vi "Main.vi"() -> ()   [LabVIEW 2013]
doc: "This template is for the Queued Message Handler design pattern.\n\nThe Event Handling Loop generates messages based on user interface actions.\n\nThe Message Handling Loop processes messages generated by the Event Handling Loop, or by other messages. The messages are string values, so new messages can be added easily to the Message Cases case structure in the Message Handling Loop. Each message cluster can also provide an optional value for Message Data, which is a variant that can be converted to whatever message-specific data is required."
uses:
  <vilib>/vision/Image Controls.llb/IMAQ Image.ctl
  Image Processing/Mask ROI FG Enum.ctl
  Message Passing/MsgQ Loops enum.ctl
  System Status/Status FG Enum.ctl
  Globals/Average Sector Data.vi
  controls/UI Data.ctl
  Message Queue/Message Queue.lvlib
  User Event - Stop/User Event - Stop.lvlib
  FPGA/FPGA Frame Grabbing.lvlib
  Image Processing/Image Processing.lvlib
  Common/State Machines/State Machine Lib.lvlib
  Message Passing/Main MsgQ.lvlib
  Common/GUI/GUI.lvlib
  <vilib>/rvi/interface/nirviReadWriteControl/nirviReadWriteControl.xnode
  FGs/FPGA_Reference.ctl
  FPGA Bitfiles/WBA256SectorsSim_FPGATargetSim.lvbitx
  <vilib>/rvi/errors/niLvFpgaMergeErrorWithErrorCode.vi
  NiFpgaLv.dll
  <vilib>/rvi/errors/niLvFpgaAdjustHostInterfaceError.vi
panel:
  out "Frame Count":u16
  out "Frames Acquired":u32
  in  "Disable Background Subtraction":bool
  out "Analysis Ticks":u32
  out "Accumulate Ticks":u32
  out "FPGA Display Image":T1(plugin-control)
  out "Right Wingbeat Avg Graph":u8[](graph)
  in  "Start Serial Server":bool=TRUE
  out "Left Wingbeat Avg Graph":u8[](graph)
  in  "Stop Charts":bool
  in  "Wing ROIs":T2
  out "FPGA image info":T5={"Image Type"=0, "Unit"=enum."Undefined", "X Resolution"=2040, "Y Resolution"=1088, "X Step"=1.0, "Y Step"=1.0, "Image Name"="Image"} {"Image Type" items=["Grayscale (U8)", "Grayscale (I16)", "Grayscale (SGL)", "Complex (CSG)", "RGB (U32)", "HSL (U32)", "RGB (U64)", "Grayscale (U16)"]}
  in  "Stream?":bool
  out "FPGA Image":T1
  in  "Test Visual Response":bool
  in  "Test FPGA":bool
  out "Status Update":string="VI Stopped"
  in  "Define Mask":bool
  in  "Acquire Image":bool
  in  "Stop":bool
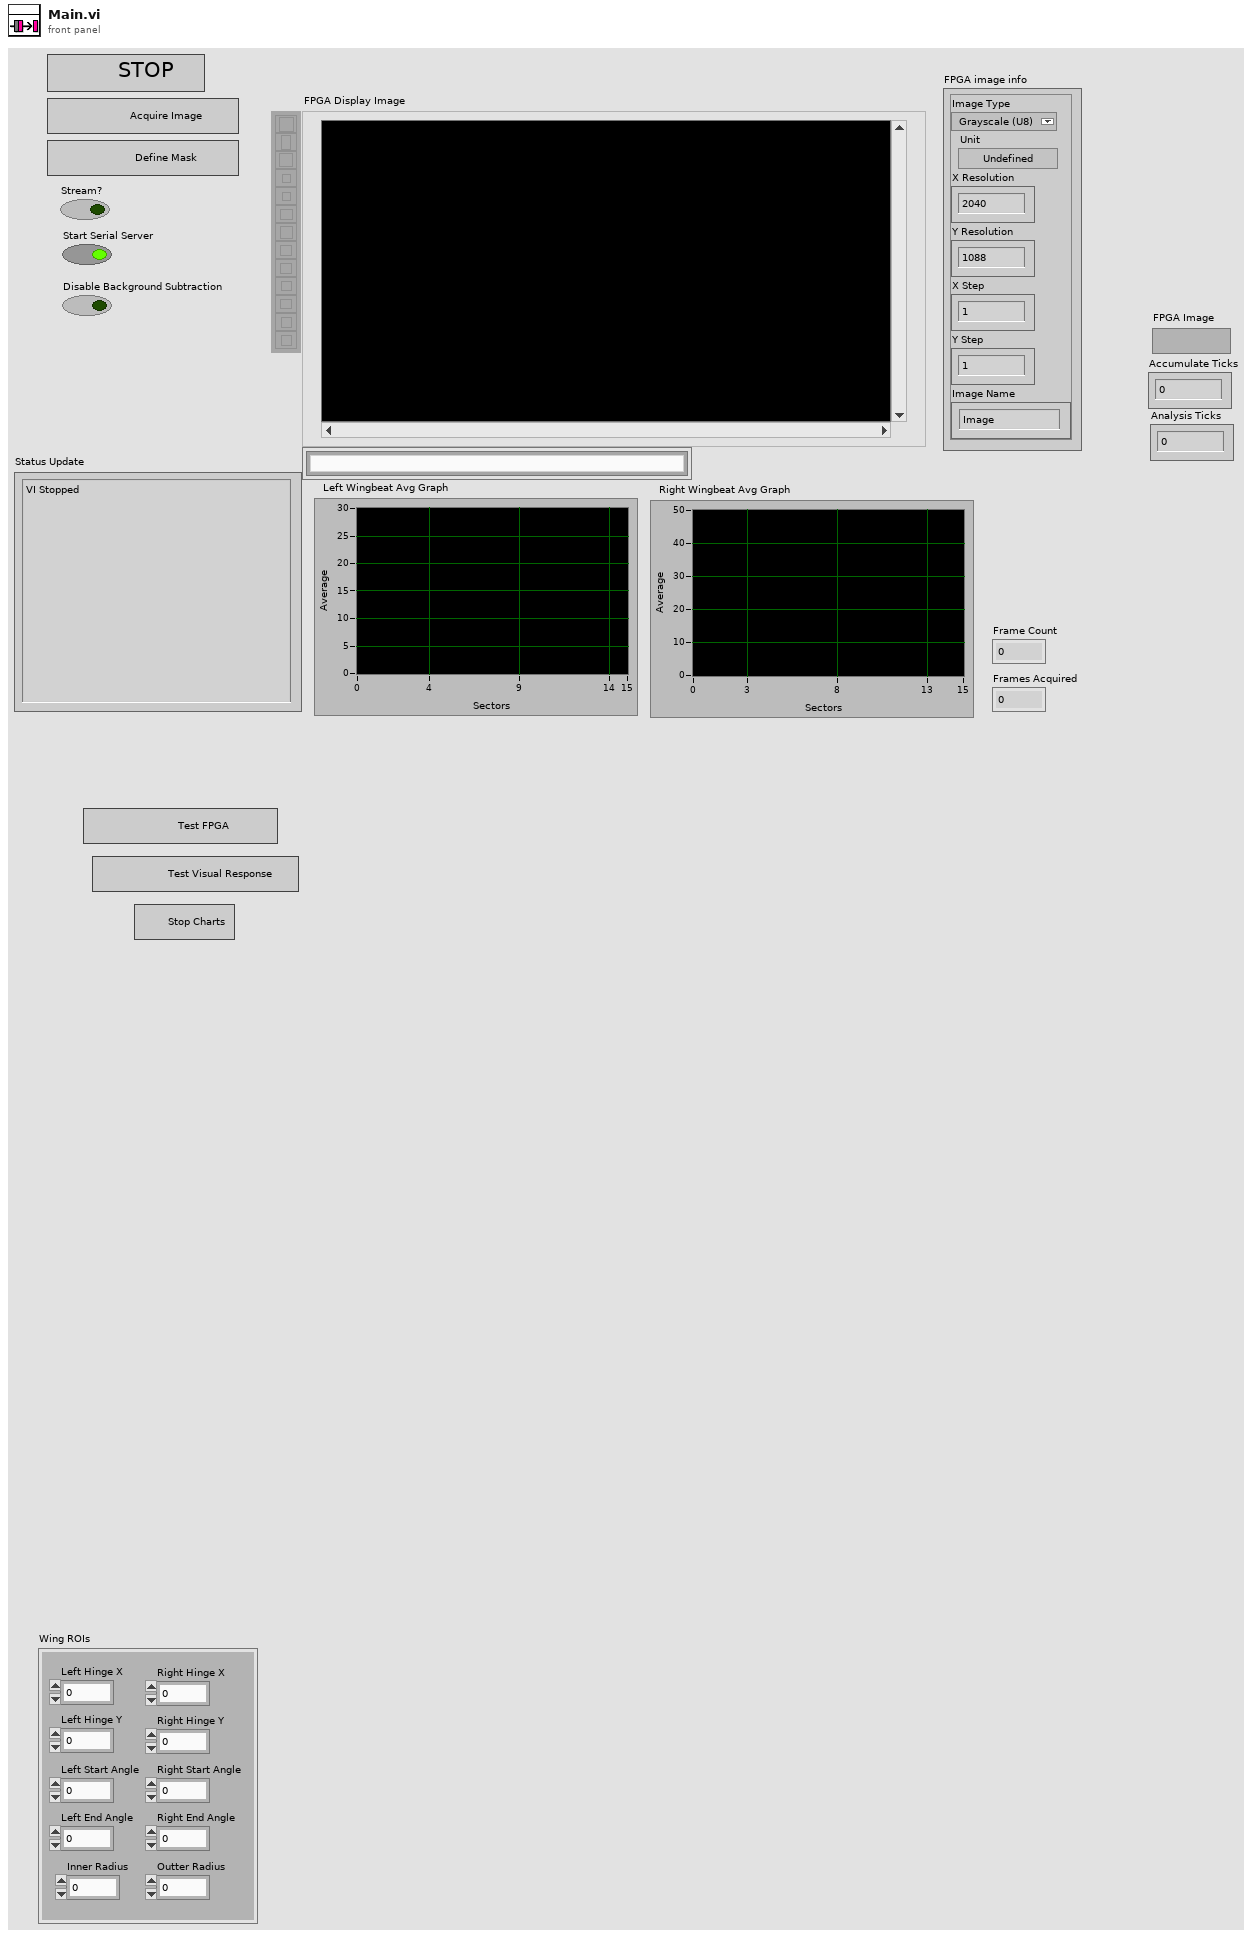
[diagram p1: front panel]
types:
  T1 = typedef "IMAQ Image.ctl" = refnum<image>
  T2 = cluster{"Left Hinge X":u16, "Left Hinge Y":u16, "Inner Radius":u16, "Outter Radius":u16, "Right Hinge X":u16, "Right Hinge Y":u16, "Right Start Angle":i16, "Right End Angle":i16, "Left Start Angle":i16, "Left End Angle":i16}
  T3 = typedef "Image Type" = u32
  T4 = typedef "Image Unit" = enum32{"Undefined", "Angström", "Micrometer", "Millimeter", "Centimeter", "Meter", "Kilometer", "Microinch", "Inch", "Feet", "Nautical miles", "Standard miles", "Steps"}
  T5 = cluster{"Image Type":T3, "Unit":T4, "X Resolution":i32, "Y Resolution":i32, "X Step":sgl, "Y Step":sgl, "Image Name":string}
  T6 = typedef "State Machine Lib.lvlib/STATE cluster.ctl" = cluster{"State":string, "Parameters":variant}
  T7 = typedef "Main MsgQ.lvlib/MsgQ Loops enum.ctl" = enum16{"User Interface", "Image Acq"}
  T8 = typedef "Mask ROI FG Enum.ctl" = enum16{"Read", "Write", "Enable Background", "Disable Background"}
  T9 = typedef "Status FG Enum.ctl" = enum16{"Reset", "Read", "Write"}
  T10 = typedef "FPGA_Reference.ctl" = refnum<k20>
  T11 = typedef "Mask ROI Cluster.ctl" = cluster{"left annulus":T12, "right annulus":T12, "Threshold Range":cluster{"Lower value":dbl, "Upper value":dbl}, "[Avg BG]":u8[], "Number of Sectors":u8, "Left ROI":T13, "Right ROI":T13, "Left Start Angle Duty Cycle":fxp<+,8,0>, "Left End Angle Duty Cycle":fxp<+,8,0>, "Right End Angle Duty Cycle":fxp<+,8,0>, "Right Start Angle Duty Cycle":fxp<+,8,0>, "[Sector ROIs]":T13[]}
  T12 = typedef "IMAQ Circle" = cluster{"Center X":i32, "Center Y":i32, "Inner Radius":i32, "Outer Radius":i32, "Start Angle":dbl, "End Angle":dbl}
  T13 = typedef "ROI Descriptor" = cluster{"Global Rectangle":i32[], "Contours":cluster{"ID":enum32{"External", "Internal"}, "Type":u32, "Coordinates":i32[]}[]}
  T14 = typedef "UI Data.ctl" = cluster{"Boolean <Replace Me>":bool, "Initial Message":string, "Numeric <Replace Me>":dbl, "Acquire Image Ref":refnum<vi>, "Define Mask Ref":refnum<vi>, "Status Update Ref":refnum<vi>, "Stop Button Ref":refnum<vi>, "FPGA Image":T1, "Processed Image":T1, "Left Annulus":cluster{"Center X":i32, "Center Y":i32, "Inner Radius":i32, "Outer Radius":i32, "Start Angle":dbl, "End Angle":dbl}, "Right Annulus":cluster{"Center X":i32, "Center Y":i32, "Inner Radius":i32, "Outer Radius":i32, "Start Angle":dbl, "End Angle":dbl}}
  T15 = typedef "Message Queue.lvlib/All Message Queues.ctl" = cluster{"UI":refnum<queue>}
  T16 = cluster{"Center X":i32, "Center Y":i32, "Inner Radius":i32, "Outer Radius":i32, "Start Angle":dbl, "End Angle":dbl}
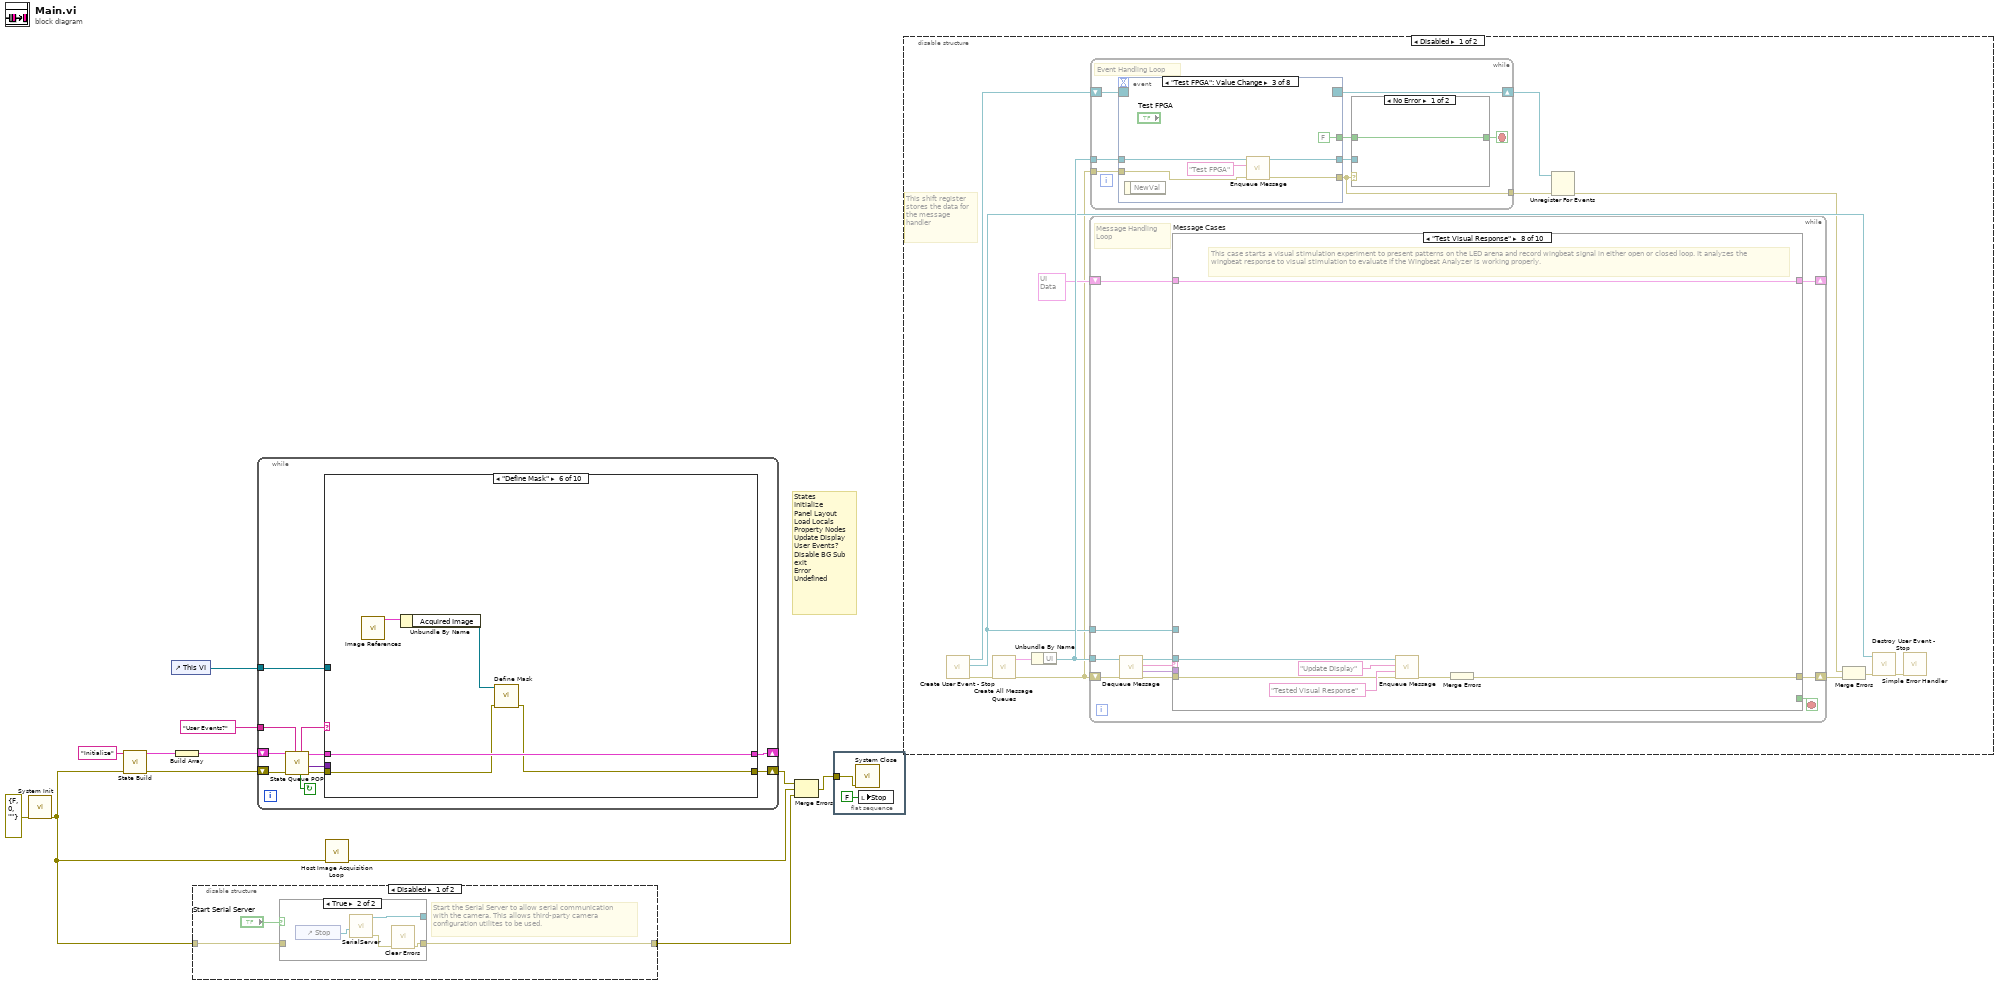
[diagram p0: block diagram]
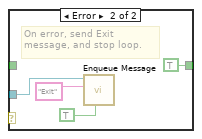
[diagram p4: hidden frame]
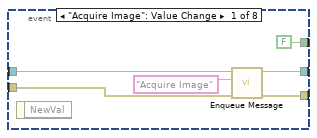
[diagram p5: hidden frame]
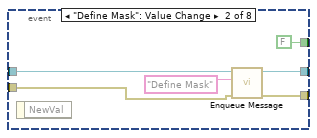
[diagram p6: hidden frame]
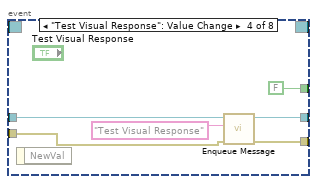
[diagram p7: hidden frame]
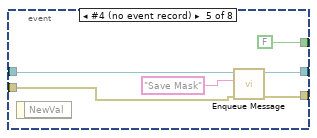
[diagram p8: hidden frame]
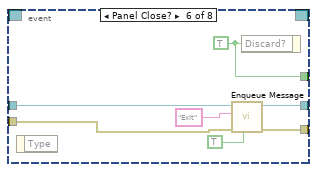
[diagram p9: hidden frame]
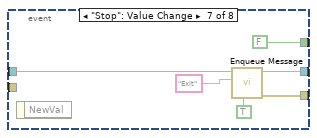
[diagram p10: hidden frame]
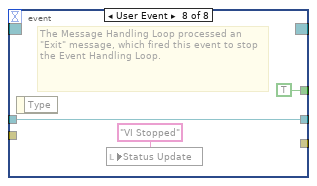
[diagram p11: hidden frame]
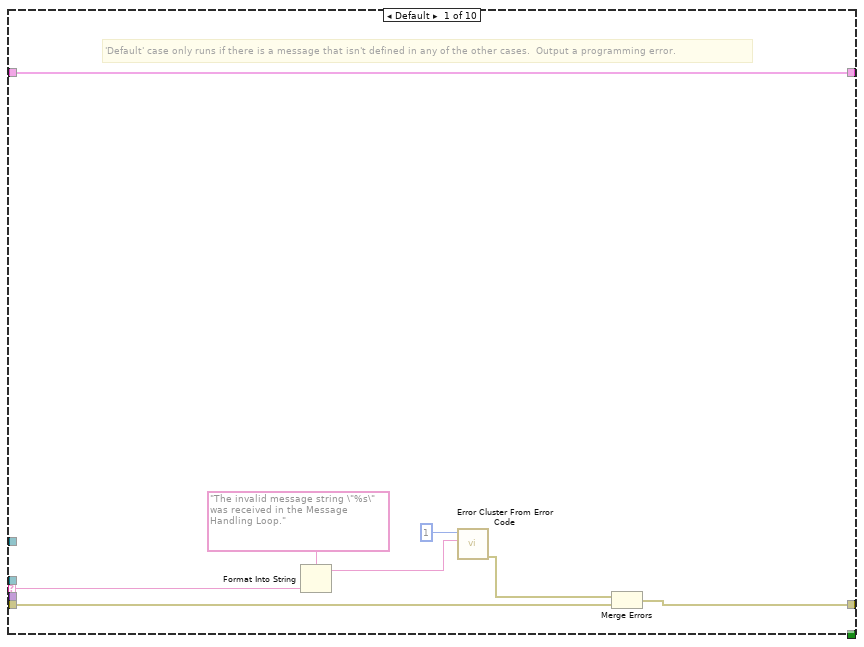
[diagram p12: hidden frame]
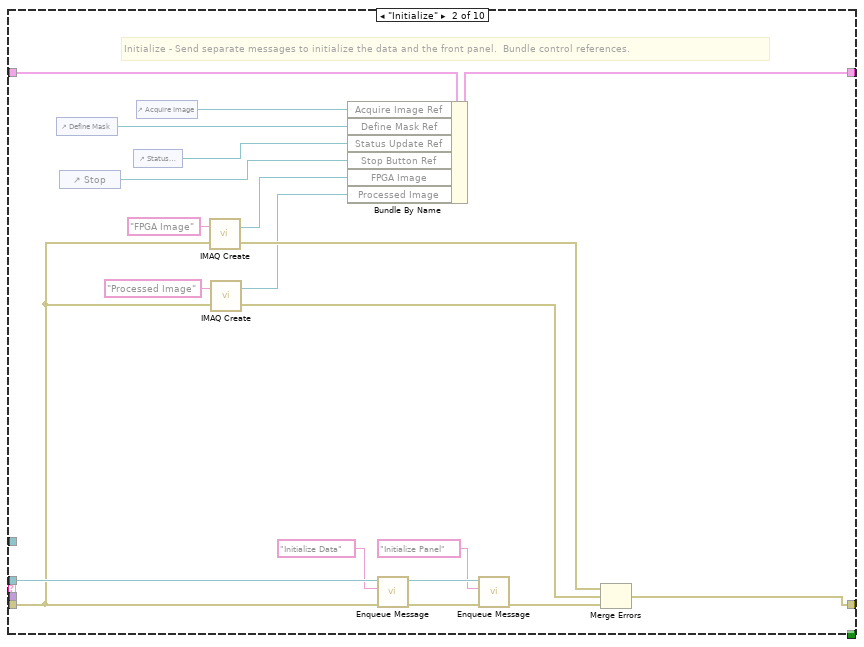
[diagram p13: hidden frame]
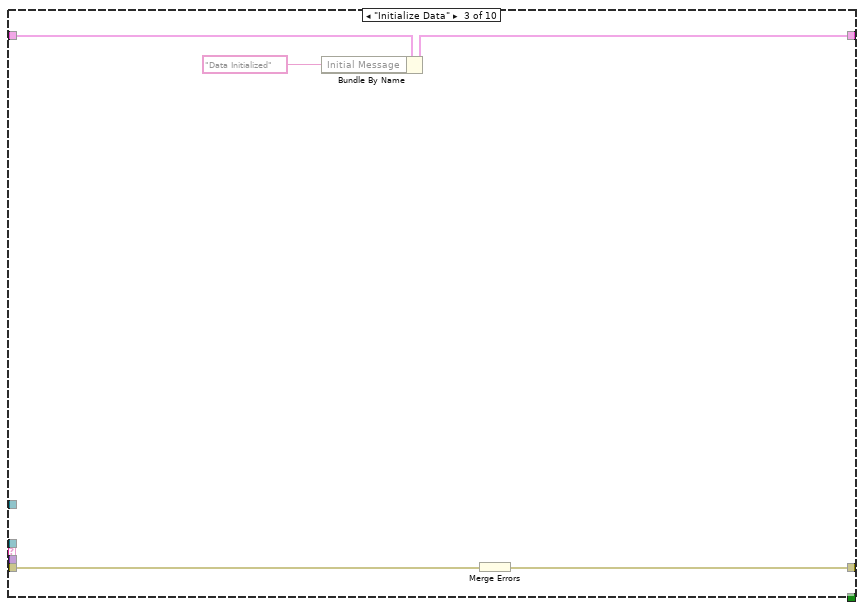
[diagram p14: hidden frame]
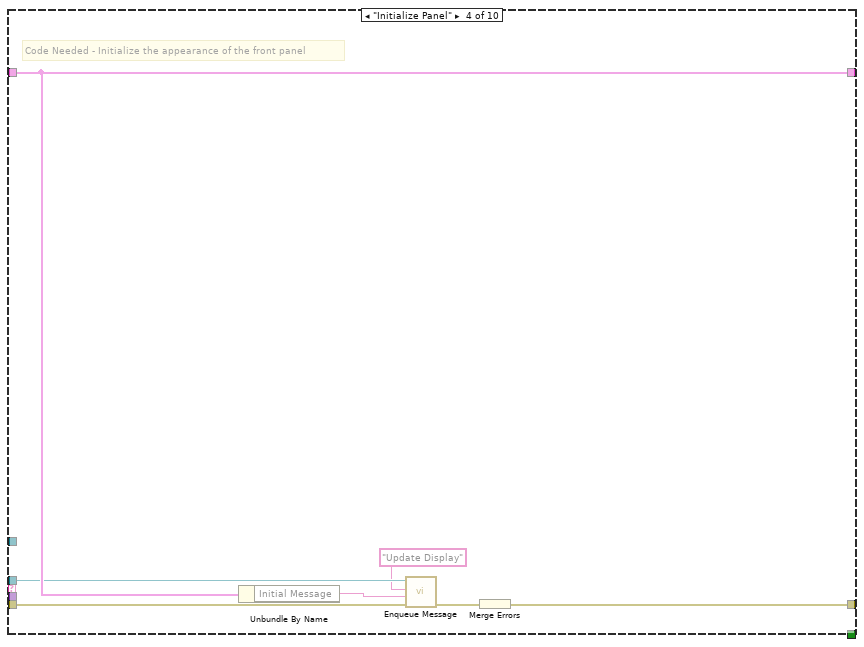
[diagram p15: hidden frame]
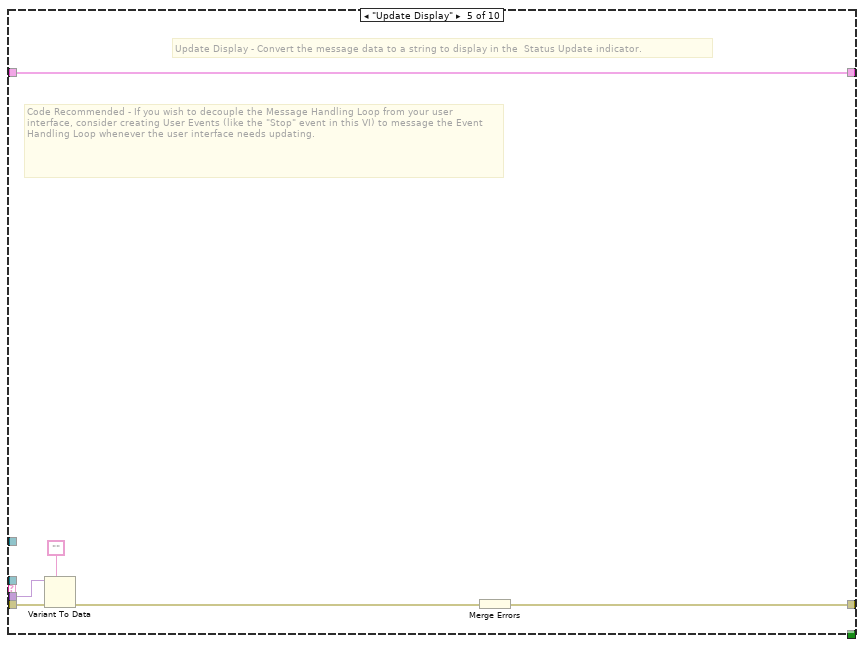
[diagram p16: hidden frame]
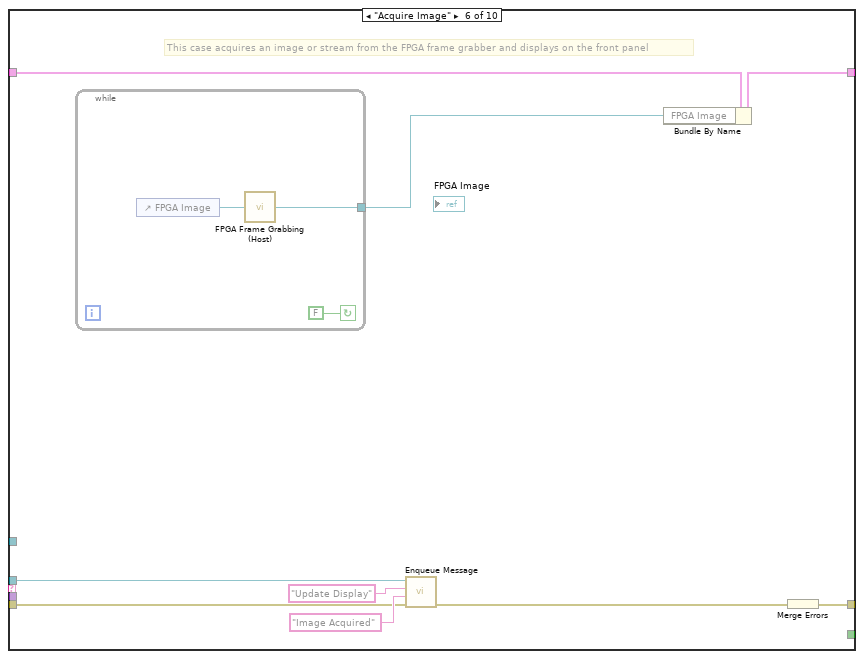
[diagram p17: hidden frame]
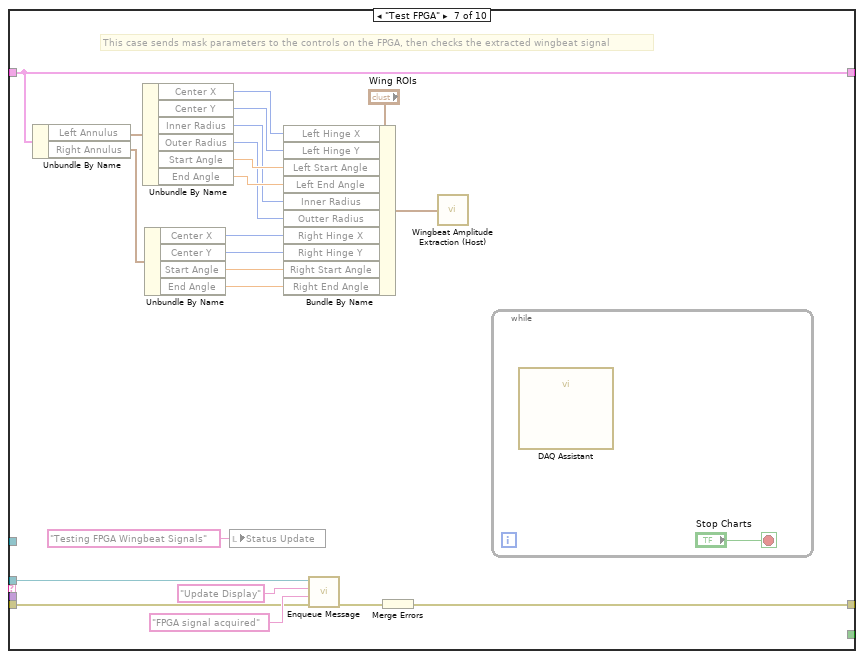
[diagram p18: hidden frame]
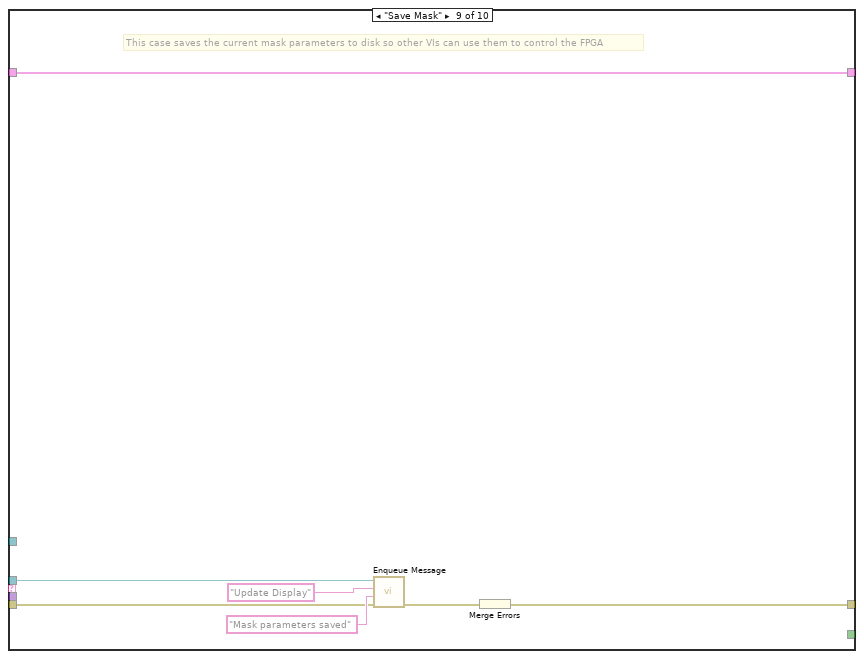
[diagram p19: hidden frame]
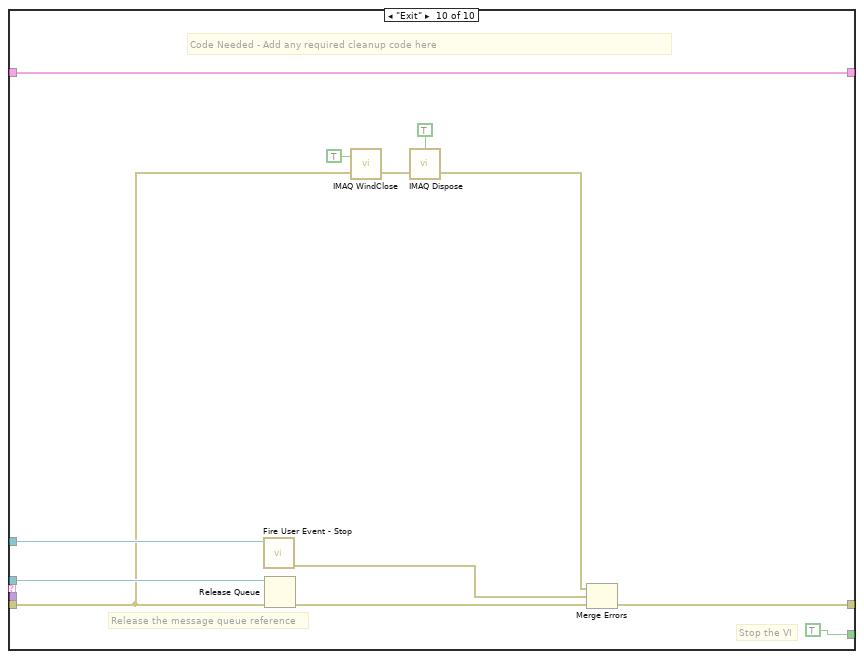
[diagram p20: hidden frame]
diagram:
  # "States\nInitialize\nPanel Layout\nLoad Locals\nProperty Nodes\nUpdate Display\nUser Events?\nDisable BG Sub\nexit\nError\nUndefined"
  n1 = call "System Init.vi"("error in (no error)"=errorcluster {"status"=FALSE, "code"=0, "source"=""}) -> ("error out"=w11:errorcluster)  [unwired: 10 in]
  n2 = call "State Build.vi"("error in (no error)"=w11, "State"="Initialize") -> ("error out"=w7:errorcluster, "State Out"=w9:T6)  [unwired: 8 in]
  n3 = control-ref of="This VI"() -> (w5:refnum<vi>)
  n4 = Build Array(w9) -> (w8:T6[])
  n5 = disable-structure shown="Disabled" {
    disable-tunnel: w11 -> [w14 w21]
    disable-tunnel: [w13 w21] -> w1
    frame Disabled {
      # "Start the Serial Server to allow serial communication\nwith the camera. This allows third-party camera\nconfiguration utilites to be used."
      n6 = case shown="True" "Start Serial Server" {
        tunnel: [_ w20] -> _
        tunnel: w14 -> [w16 _]
        tunnel: [w16 w18] -> w13
        frame False {
        }
        frame True {
          n7 = control-ref of="Stop"() -> (w19:refnum<vi>)
          n8 = call "SerialServer.vi"("Stop Refnum"=w19) -> ("error out"=w17:errorcluster, "FPGA VI Reference Out"=w20:refnum<k20>)  [unwired: 5 in]
          n9 = call <vilib>:"Clear Errors.vi"("error in (no error)"=w17) -> ("error out"=w18:errorcluster)  [unwired: 6 in]
        }
      }
    }
    frame Enabled {
    }
  }
  n10 = while {
    shift-right: [w26] -> _
    shift-left: w8 -> [w32]
    shift-right: [w24] -> w4
    shift-left: w7 -> [w31]
    tunnel: "User Events?" ("State") -> [w29]
    tunnel: w5 -> [w27]
    stop <- w30 continue-if-true
    n11 = call "State Queue POP.vi"("Default state"=w29, "error in (no error)"=w31, "State que in"=w32) -> ("error out"=w23:errorcluster, "Parameters"=w22:variant, "State que out"=w25:T6[], "Not Exit?"=w30:bool, "State case out"=w28:string)  [unwired: 4 in]
    n12 = case shown="\"Define Mask\"" w28 {
      tunnel: w27 -> [_ _ w43 _ _ _ _ _ _ _]
      tunnel: [w34 w35 w40 w46 w48 w53 w54 w71 w112 w140] -> w26
      tunnel: w25 -> [w34 w38 w40 w46 w48 w53 w54 w70 _ w140]
      tunnel: [w33 w36 w41 w45 w47 w51 w55 w69 w111 w138] -> w24
      tunnel: w23 -> [w33 w37 w42 w45 w47 w52 w66 w68 w113 w122]
      tunnel: w22 -> [_ _ _ _ _ _ w65 w67 _ _]
      frame Default {
      }
      frame "Initialize" {
        n13 = call "State Queue PUSH multiple states no parameters.vi"("States to queue"=string[] ["Panel Layout", "Load Locals", "Property Nodes", "Update Display"], "error in (no error)"=w37, "State que in"=w38) -> ("error out"=w36:errorcluster, "State que out"=w35:T6[])  [unwired: 7 in]
      }
      frame "Panel Layout" {
        # "Reset origin to 0,0"
        n14 = call "Reset all pane origins.vi"("error in (no error"=w42, "Vi Ref In"=w43) -> ("error out"=w41:errorcluster)  [unwired: 8 in, 1 out]
      }
      frame "Load Locals" {
        w44 = FALSE ("Stream?")
        n15 = local write "Stream?"(w44) -> ()
        n16 = local write "Disable Background Subtraction"(w44) -> ()
      }
      frame "Property Nodes" {
      }
      frame "Define Mask" {
        n17 = call "Image References.vi"() -> ("Images"=w50:cluster{"Acquired Image":T1, "Display Image":T1})  [unwired: 10 in, 1 out]
        n18 = Unbundle By Name(w50) -> ("Acquired Image"=w49:T1)
        n19 = call "Define Mask.vi"("error in (no error)"=w52, "FPGA Image"=w49) -> ("error out"=w51:errorcluster)  [unwired: 9 in]
      }
      frame "Disable BG Sub" {
        n20 = Variant To Data(error in=w66, type=FALSE, Variant=w65) -> (data=w63:bool, error out=w60:errorcluster)
        n21 = Select(t=Mask_ROI_FG_Enum."Disable Background" ("Operation"), s=w63, f=Mask_ROI_FG_Enum."Enable Background" ("Operation")) -> (s? t:f=w59:T8)
        n22 = call "Mask ROI FG.vi"("error in (no error)"=w60, "Operation"=w59) -> ("error out"=w56:errorcluster)  [unwired: 8 in, 1 out]
        n23 = call "Send MsgQ.vi"("error in (no error)"=w56, "Message String"="Update Sector Parameters", "Send to MsgQ"=MsgQ_Loops_enum."Image Acq") -> ("error out"=w55:errorcluster)  [unwired: 8 in]
      }
      frame "User Events?" {
        n24 = event shown="[1] \"Acquire Image\": Value Change" {
          selector: _ -> [_ _ _ _ _ _]
          dyn-events: _ -> [_ _ _ _ _ _]
          timeout: 200 -> [_ _ _ _ _ _]
          tunnel: [w74 w87 w90 w97 w103 w106] -> w71
          tunnel: w70 -> [w75 w87 w90 w99 w105 w109]
          tunnel: [w76 w84 w91 w96 w102 w107] -> w69
          tunnel: w68 -> [w77 w85 w92 w98 w104 w108]
          tunnel: w67 -> [_ _ _ _ _ _]
          event Timeout {
            n25 = event-data() -> ()  [unwired: 1 in, 3 out]
            n26 = disable-structure shown="Disabled" {
              frame Disabled {
                n27 = call "FPGA Reference FG.vi"() -> ("FPGA VI Reference Out"=w80:T10)  [unwired: 11 in]
                n28 = xnode "Read/Write Control"("FPGA VI Reference In"=w80) -> ("Accumulate Ticks"=→"Accumulate Ticks", "Analysis Ticks"=→"Analysis Ticks":u32)  [unwired: 1 in, 2 out]
              }
              frame Enabled {
              }
            }
            n29 = call "State Queue PUSH.vi"("State case"="Update Display", "error in (no error)"=w77, "State que in"=w75) -> ("error out"=w76:errorcluster, "State que out"=w74:T6[])  [unwired: 7 in]
          }
          event "Acquire Image": Value Change {
            n30 = event-data() -> ()  [unwired: 1 in, 6 out]
            n31 = feedback #1(u16 0 ("Frame Count")) -> (w82:u16)
            n32 = call "Send MsgQ.vi"("error in (no error)"=w85, "Message String"="Acquire Single Image", "Send to MsgQ"=MsgQ_Loops_enum."Image Acq") -> ("error out"=w84:errorcluster)  [unwired: 8 in]
            n33 = Increment(x=w82) -> (x+1=w81:u16)
            "Frame Count" <- w81
            n34 = feedback-in #1(w81) -> ()
          }
          event "Stream?": Value Change {
            n35 = event-data() -> ("NewVal"=w89:bool)  [unwired: 1 in, 5 out]
            n36 = call "Send MsgQ.vi"("error in (no error)"=w92, "Data In"=w89, "Message String"="Stream Image", "Send to MsgQ"=MsgQ_Loops_enum."Image Acq") -> ("error out"=w91:errorcluster)  [unwired: 7 in]
          }
          event "Define Mask": Value Change {
            n37 = event-data() -> ()  [unwired: 1 in, 6 out]
            n38 = call "State Queue PUSH.vi"("State case"="Define Mask", "error in (no error)"=w98, "State que in"=w99) -> ("error out"=w96:errorcluster, "State que out"=w97:T6[])  [unwired: 7 in]
          }
          event "Disable Background Subtraction": Value Change {
            n39 = event-data() -> ("NewVal"=w100:bool)  [unwired: 1 in, 5 out]
            n40 = call "State Queue PUSH.vi"("State case"="Disable BG Sub", "error in (no error)"=w104, "Parameters"=w100, "State que in"=w105) -> ("error out"=w102:errorcluster, "State que out"=w103:T6[])  [unwired: 6 in]
          }
          event "Stop": Value Change {
            n41 = event-data() -> ()  [unwired: 1 in, 6 out]
            n42 = call "State Queue PUSH.vi"("State case"="exit", "error in (no error)"=w108, "State que in"=w109) -> ("error out"=w107:errorcluster, "State que out"=w106:T6[])  [unwired: 7 in]
          }
        }
      }
      frame "exit" {
        n43 = call "Broadcast Exit.vi"("error in"=w113) -> ("error out"=w111:errorcluster)  [unwired: 10 in]
        n44 = call "Queue EXIT state.vi"() -> ("Exit State Q"=w112:T6[])  [unwired: 1 in]
      }
      frame "Update Display" {
        n45 = call "Image References.vi"() -> ("Images"=w118:cluster{"Acquired Image":T1, "Display Image":T1})  [unwired: 10 in, 1 out]
        n46 = call "Status FG.vi"("Operation"=Status_FG_Enum."Read") -> ("Status Out"=→"Status Update":string)  [unwired: 9 in, 1 out]
        n47 = call "Mask ROI FG.vi"("Operation"=Mask_ROI_FG_Enum."Read") -> ("Mask ROI Out"=w135:T11)  [unwired: 9 in, 1 out]
        n48 = Unbundle By Name(w118) -> ("Acquired Image"=w117:T1, "Display Image"=w116:T1)
        n49 = Unbundle By Name(w135) -> ("Number of Sectors"=w132:u8)
        n50 = global read "Average Sector Data.vi" "# of Frames Acquired"() -> (→"Frames Acquired":u32)
        n51 = global read "Average Sector Data.vi" "[Average Sector Data]"() -> (w137:u8[])
        n52 = call "Overlay Image with Sector ROI.vi"("FPGA Display Image In"=w116, "error in"=w122, "FPGA Image"=w117) -> ("error out"=w121:errorcluster, "FPGA Display Image Out"=→"FPGA Display Image":T1)  [unwired: 7 in]
        n53 = call "IMAQ GetImageInfo"("error in (no error)"=w121, "Image"=w117) -> ("error out"=w139:errorcluster, "X Step"=w127:sgl, "Y Resolution"=w126:i32, "X Resolution"=w125:i32, "Y Step"=w128:sgl, "Unit"=w124:T4, "Image Name"=w129:string, "Image Type"=w123:T3)  [unwired: 2 in]
        n54 = Split 1D Array(array=w137, index=w132) -> (first subarray=→"Left Wingbeat Avg Graph":u8[], second subarray=→"Right Wingbeat Avg Graph":u8[])
        n55 = local read "FPGA image info"() -> (w131:T5)
        n56 = Bundle By Name(cluster=w131, "Image Type"=w123, "Unit"=w124, "X Resolution"=w125, "Y Resolution"=w126, "X Step"=w127, "Y Step"=w128, "Image Name"=w129) -> (→"FPGA image info":T5)
        n57 = call <vilib>:"Clear Errors.vi"("error in (no error)"=w139) -> ("error out"=w138:errorcluster)  [unwired: 6 in]
      }
    }
  }
  n58 = call "Host Image Acquisition Loop.vi"("error in"=w11) -> ("error out"=w3:errorcluster)  [unwired: 10 in]
  n59 = Merge Errors(w4, w3, w1) -> (w2:errorcluster)
  n60 = flat-sequence {
    tunnel: w2 -> [w142]
    frame #0 {
      n61 = call "System Close.vi"("error in (no error)"=w142) -> ()  [unwired: 10 in, 1 out]
      n62 = local write "Stop"(FALSE ("Stop")) -> ()
    }
  }
  n63 = disable-structure shown="Disabled" {
    frame Disabled {
      # "This shift register\nstores the data for the message handler"
      n64 = call "Create User Event - Stop.vi"() -> ("error out"=w151:errorcluster, "User Event - Stop"=w148:refnum<user-event>, "Stop Event Registration Refnum"=w152:refnum<event-registration>)  [unwired: 9 in]
      n65 = call "Create All Message Queues.vi"("error in (no error)"=w151) -> ("error out"=w143:errorcluster, "Message Queues out"=w155:T15)  [unwired: 9 in]
      n66 = Unbundle By Name(w155) -> ("UI"=w153:refnum<queue>)
      n67 = while {
        tunnel: w153 -> [w215]
        shift-right: [w224] -> _
        shift-left: T14 {"Boolean <Replace Me>"=TRUE, "Initial Message"="", "Numeric <Replace Me>"=0.0, "Acquire Image Ref"=refnum, "Define Mask Ref"=refnum, "Status Update Ref"=refnum, "Stop Button Ref"=refnum, "FPGA Image"=refnum, "Processed Image"=refnum, "Left Annulus"={"Center X"=0, "Center Y"=0, "Inner Radius"=0, "Outer Radius"=0, "Start Angle"=0.0, "End Angle"=0.0}, "Right Annulus"={"Center X"=0, "Center Y"=0, "Inner Radius"=0, "Outer Radius"=0, "Start Angle"=0.0, "End Angle"=0.0}} ("Data Cluster") -> [w225]
        tunnel: w148 -> [w221]
        shift-right: [w222] -> w154
        shift-left: w143 -> [w220]
        stop <- w223 stop-if-true
        # "Message Handling Loop"
        n68 = call "Dequeue Message.vi"("error in (no error)"=w220, "Message Queue"=w215) -> ("error out"=w219:errorcluster, "Message Data"=w217:variant, "Message"=w218:string, "dup Message Queue"=w216:refnum<queue>)  [unwired: 6 in]
        n69 = case "Message Cases" shown="\"Test Visual Response\"" w218 {
          selector: w218 -> [w231 _ _ _ _ _ _ _ _ _]
          tunnel: w216 -> [_ w251 _ w262 _ w279 w302 w310 w318 w334]
          tunnel: w219 -> [w228 w236 w258 w263 w270 w274 w303 w311 w316 w323]
          tunnel: [w226 w238 w254 w264 w271 w281 w301 w309 w321 w330] -> w222
          tunnel: w225 -> [w233 w248 w257 w265 w272 w276 w300 w315 w322 w333]
          tunnel: [w233 w247 w256 w265 w272 w275 w300 w315 w322 w333] -> w224
          tunnel: [_ _ _ _ _ _ _ _ _ TRUE] -> w223
          tunnel: w217 -> [_ _ _ _ w269 _ _ _ _ _]
          tunnel: w221 -> [_ _ _ _ _ _ _ _ _ w329]
          frame Default {
            # "'Default' case only runs if there is a message that isn't defined in any of the other cases.  Output a programming error."
            n70 = Format Into String(format string="The invalid message string \"%s\" was received in the Message Handling Loop." ("Unknown Message Error Text"), w231) -> (resulting string=w229:string)  [unwired: 2 in, 1 out]
            n71 = call <vilib>:"Error Cluster From Error Code.vi"("error message (\"\")"=w229, "error code (0)"=1) -> ("error out"=w227:errorcluster)  [unwired: 7 in]
            n72 = Merge Errors(w227, w228) -> (w226:errorcluster)
          }
          frame "Initialize" {
            # "Initialize - Send separate messages to initialize the data and the front panel.  Bundle control references."
            n73 = control-ref of="Define Mask"() -> (w245:refnum<vi>)
            n74 = control-ref of="Stop"() -> (w243:refnum<vi>)
            n75 = control-ref of="Status Update"() -> (w244:refnum<vi>)
            n76 = control-ref of="Acquire Image"() -> (w246:refnum<vi>)
            n77 = call "IMAQ Create"("Image Name"="FPGA Image", "error in (no error)"=w236) -> ("New Image"=w241:T1, "error out"=w237:errorcluster)  [unwired: 3 in]
            n78 = call "IMAQ Create"("Image Name"="Processed Image", "error in (no error)"=w236) -> ("New Image"=w234:T1, "error out"=w235:errorcluster)  [unwired: 3 in]
            n79 = Bundle By Name(cluster=w248, "Acquire Image Ref"=w246, "Define Mask Ref"=w245, "Status Update Ref"=w244, "Stop Button Ref"=w243, "FPGA Image"=w241, "Processed Image"=w234) -> (w247:T14)
            n80 = call "Enqueue Message.vi"("error in (no error)"=w236, "Message"="Initialize Data", "Message Queue"=w251) -> ("error out"=w253:errorcluster, "dup Message Queue"=w252:refnum<queue>)  [unwired: 7 in]
            n81 = call "Enqueue Message.vi"("error in (no error)"=w253, "Message"="Initialize Panel", "Message Queue"=w252) -> ("error out"=w239:errorcluster)  [unwired: 7 in, 1 out]
            n82 = Merge Errors(w237, w235, w239) -> (w238:errorcluster)
          }
          frame "Initialize Data" {
            n83 = Bundle By Name(cluster=w257, "Initial Message"="Data Initialized") -> (w256:T14)
            n84 = Merge Errors(w258) -> (w254:errorcluster)
          }
          frame "Initialize Panel" {
            # "Code Needed - Initialize the appearance of the front panel"
            n85 = Unbundle By Name(w265) -> ("Initial Message"=w259:string)
            n86 = call "Enqueue Message.vi"("error in (no error)"=w263, "Message Data"=w259, "Message"="Update Display", "Message Queue"=w262) -> ("error out"=w261:errorcluster)  [unwired: 6 in, 1 out]
            n87 = Merge Errors(w261) -> (w264:errorcluster)
          }
          frame "Update Display" {
            # "Code Recommended - If you wish to decouple the Message Handling Loop from your user interface, consider creating User Events (like the \"Stop\" event in this VI) to message the Event Handling Loop whenever the user interface needs updating."
            # "Update Display - Convert the message data to a string to display in the  Status Update indicator."
            n88 = Variant To Data(error in=w270, type="", Variant=w269) -> (data=w266:string, error out=w267:errorcluster)
            n89 = Merge Errors(w267) -> (w271:errorcluster)
          }
          frame "Acquire Image" {
            # "This case acquires an image or stream from the FPGA frame grabber and displays on the front panel"
            n90 = while {
              tunnel: [w284] -> w273
              stop <- FALSE continue-if-true
              n91 = control-ref of="FPGA Image"() -> (w283:refnum<vi>)
              n92 = call "FPGA Frame Grabbing (Host).vi"("Ctl Refnum"=w283) -> ("Image"=w284:T1)
            }
            n93 = call "Enqueue Message.vi"("error in (no error)"=w274, "Message Data"="Image Acquired" ("\"Do Something\" button pressed"), "Message"="Update Display", "Message Queue"=w279) -> ("error out"=w280:errorcluster)  [unwired: 6 in, 1 out]
            n94 = Bundle By Name(cluster=w276, "FPGA Image"=w273) -> (w275:T14)
            n95 = Merge Errors(w280) -> (w281:errorcluster)
          }
          frame "Test FPGA" {
            # "This case sends mask parameters to the controls on the FPGA, then checks the extracted wingbeat signal"
            n96 = Unbundle By Name(w300) -> ("Left Annulus"=w299:T16, "Right Annulus"=w298:T16)
            n97 = Unbundle By Name(w299) -> ("Center X"=w296:i32, "Center Y"=w295:i32, "Inner Radius"=w292:i32, "Outer Radius"=w291:i32, "Start Angle"=w294:dbl, "End Angle"=w293:dbl)
            n98 = Unbundle By Name(w298) -> ("Center X"=w290:i32, "Center Y"=w289:i32, "Start Angle"=w288:dbl, "End Angle"=w287:dbl)
            n99 = local write "Status Update"("Testing FPGA Wingbeat Signals" ("Status Update")) -> ()
            n100 = Bundle By Name(cluster="Wing ROIs", "Left Hinge X"=w296, "Left Hinge Y"=w295, "Left Start Angle"=w294, "Left End Angle"=w293, "Inner Radius"=w292, "Outter Radius"=w291, "Right Hinge X"=w290, "Right Hinge Y"=w289, "Right Start Angle"=w288, "Right End Angle"=w287) -> (w286:T2)
            n101 = call "Enqueue Message.vi"("error in (no error)"=w303, "Message Data"="FPGA signal acquired" ("\"Do Something\" button pressed"), "Message"="Update Display", "Message Queue"=w302) -> ("error out"=w306:errorcluster)  [unwired: 6 in, 1 out]
            n102 = Merge Errors(w306) -> (w301:errorcluster)
            n103 = call "Wingbeat Amplitude Extraction (Host).vi"("Wing ROIs"=w286) -> ()  [unwired: 1 in]
            n104 = while {
              stop <- "Stop Charts" stop-if-true
              n105 = call "DAQ Assistant"() -> ("data"=w307:dynamicdata)  [unwired: 17 in, 2 out]
            }
          }
          frame "Test Visual Response" {
            # "This case starts a visual stimulation experiment to present patterns on the LED arena and record wingbeat signal in either open or closed loop. It analyzes the wingbeat response to visual stimulation to evaluate if the Wingbeat Analyzer is working properly."
            n106 = call "Enqueue Message.vi"("error in (no error)"=w311, "Message Data"="Tested Visual Response" ("\"Do Something\" button pressed"), "Message"="Update Display", "Message Queue"=w310) -> ("error out"=w314:errorcluster)  [unwired: 6 in, 1 out]
            n107 = Merge Errors(w314) -> (w309:errorcluster)
          }
          frame "Save Mask" {
            # "This case saves the current mask parameters to disk so other VIs can use them to control the FPGA"
            n108 = call "Enqueue Message.vi"("error in (no error)"=w316, "Message Data"="Mask parameters saved" ("\"Do Something Else\" button pressed"), "Message"="Update Display", "Message Queue"=w318) -> ("error out"=w317:errorcluster)  [unwired: 6 in, 1 out]
            n109 = Merge Errors(w317) -> (w321:errorcluster)
          }
          frame "Exit" {
            # "Stop the VI"
            # "Release the message queue reference"
            # "Code Needed - Add any required cleanup code here"
            n110 = call "Fire User Event - Stop.vi"("User Event - Stop"=w329) -> ("error out"=w328:errorcluster)  [unwired: 10 in]
            n111 = Release Queue(queue=w334, error in (no error)=w323) -> (error out=w331:errorcluster)  [unwired: 1 in, 2 out]
            n112 = call "IMAQ WindClose"("Close All Windows (False)"=TRUE, "error in (no error)"=w323) -> ("error out"=w325:errorcluster)  [unwired: 4 in]
            n113 = call "IMAQ Dispose"("All Images? (No)"=TRUE, "error in (no error)"=w325) -> ("error out"=w324:errorcluster)  [unwired: 4 in]
            n114 = Merge Errors(w324, w328, w331) -> (w330:errorcluster)
          }
        }
      }
      n115 = while {
        tunnel: w153 -> [w163]
        tunnel: [w159] -> w146
        shift-right: [w157] -> w145
        shift-left: w152 -> [w158]
        tunnel: w143 -> [w156]
        stop <- w161 stop-if-true
        # "Event Handling Loop"
        n116 = event shown="[2] \"Test FPGA\": Value Change" {
          selector: w158 -> [_ _ _ _ _ _ _ _]
          dyn-events: [_ _ _ _ _ _ _ _] -> w157
          timeout: _ -> [_ _ _ _ _ _ _ _]
          tunnel: [FALSE ("Discard?") FALSE ("Discard?") FALSE ("Discard?") FALSE ("Discard?") FALSE ("Discard?") w205 FALSE ("Discard?") TRUE ("Discard?")] -> w162
          tunnel: w163 -> [w174 w180 w186 w191 w196 w204 w211 w214]
          tunnel: [w173 w178 w183 w188 w193 w203 w210 _] -> w159
          tunnel: [w172 w179 w182 w190 w195 w202 w208 w214] -> w160
          tunnel: w156 -> [w170 w176 w184 w187 w194 w199 _ _]
          event "Acquire Image": Value Change {
            n117 = event-data() -> ()  [unwired: 1 in, 1 out]
            n118 = call "Enqueue Message.vi"("error in (no error)"=w170, "Message"="Acquire Image", "Message Queue"=w174) -> ("error out"=w173:errorcluster, "dup Message Queue"=w172:refnum<queue>)  [unwired: 7 in]
          }
          event "Define Mask": Value Change {
            n119 = event-data() -> ()  [unwired: 1 in, 1 out]
            n120 = call "Enqueue Message.vi"("error in (no error)"=w176, "Message"="Define Mask", "Message Queue"=w180) -> ("error out"=w178:errorcluster, "dup Message Queue"=w179:refnum<queue>)  [unwired: 7 in]
          }
          event "Test FPGA": Value Change {
            n121 = event-data() -> ()  [unwired: 1 in, 1 out]
            n122 = call "Enqueue Message.vi"("error in (no error)"=w184, "Message"="Test FPGA", "Message Queue"=w186) -> ("error out"=w183:errorcluster, "dup Message Queue"=w182:refnum<queue>)  [unwired: 7 in]
          }
          event "Test Visual Response": Value Change {
            n123 = event-data() -> ()  [unwired: 1 in, 1 out]
            n124 = call "Enqueue Message.vi"("error in (no error)"=w187, "Message"="Test Visual Response", "Message Queue"=w191) -> ("error out"=w188:errorcluster, "dup Message Queue"=w190:refnum<queue>)  [unwired: 7 in]
          }
          event #4 (no event record) {
            n125 = event-data() -> ()  [unwired: 1 in, 1 out]
            n126 = call "Enqueue Message.vi"("error in (no error)"=w194, "Message"="Save Mask", "Message Queue"=w196) -> ("error out"=w193:errorcluster, "dup Message Queue"=w195:refnum<queue>)  [unwired: 7 in]
          }
          event Panel Close? {
            w205 = TRUE ("Discard?")
            n127 = event-data() -> ()  [unwired: 1 in, 1 out]
            n128 = call "Enqueue Message.vi"("Priority Message? (F)"=TRUE, "error in (no error)"=w199, "Message"="Exit", "Message Queue"=w204) -> ("error out"=w203:errorcluster, "dup Message Queue"=w202:refnum<queue>)  [unwired: 6 in]
            n129 = event-data("Discard?"=w205) -> ()  [unwired: 1 in, 1 out]
          }
          event "Stop": Value Change {
            n130 = event-data() -> ()  [unwired: 1 in, 1 out]
            n131 = call "Enqueue Message.vi"("Priority Message? (F)"=TRUE, "Message"="Exit", "Message Queue"=w211) -> ("error out"=w210:errorcluster, "dup Message Queue"=w208:refnum<queue>)  [unwired: 7 in]
          }
          event User Event {
            # "The Message Handling Loop processed an \"Exit\" message, which fired this event to stop the Event Handling Loop."
            n132 = event-data() -> ()  [unwired: 1 in, 1 out]
            n133 = local write "Status Update"("VI Stopped" ("VI Stopped")) -> ()
          }
        }
        n134 = case shown="No Error" w159 {
          tunnel: [w164 TRUE ("Discard?")] -> w161
          tunnel: w162 -> [w164 _]
          tunnel: w160 -> [_ w167]
          frame No Error {
          }
          frame Error {
            # "On error, send Exit message, and stop loop."
            n135 = call "Enqueue Message.vi"("Priority Message? (F)"=TRUE, "Message"="Exit", "Message Queue"=w167) -> ()  [unwired: 7 in, 2 out]
          }
        }
      }
      n136 = Unregister For Events(event registration refnum=w145, error in=w146) -> (error out=w147:errorcluster)
      n137 = Merge Errors(w147, w154) -> (w149:errorcluster)
      n138 = call "Destroy User Event - Stop.vi"("error in (no error)"=w149, "User Event - Stop"=w148) -> ("error out"=w150:errorcluster)  [unwired: 9 in]
      n139 = call <vilib>:"Simple Error Handler.vi"("error in (no error)"=w150) -> ()  [unwired: 4 in, 5 out]
    }
    frame Enabled {
    }
  }
